vi "Untitled 4.vi"() -> ()   [LabVIEW 2023]
uses:
  Control 3.ctl
panel:
  in  "Enum":T1
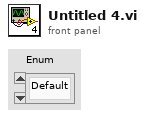
[diagram p1: front panel]
types:
  T1 = typedef "Control 3.ctl" = enum16{"Default", "PathLoaded", "RawImageLoaded", "LoadFile", "EditImage", "ImageEdited", "CloseAll"}
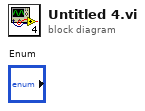
[diagram p0: block diagram]
diagram:
